vi "test_vi_new.vi"(5 "OutputReport_in":u8[](array[numeric]), 6 "DevDet_in":i32, 7 "InputReport_in":u8[](array[numeric])) -> (0 "DevDet_out":i32, 1 "OutputReport_out":u8[](array[numeric]), 2 "InputReport_out":u8[](array[numeric]) format="%x", 3 "output param":string)   [LabVIEW 2022 SP3]
uses:
  adcDLL_0001.dll
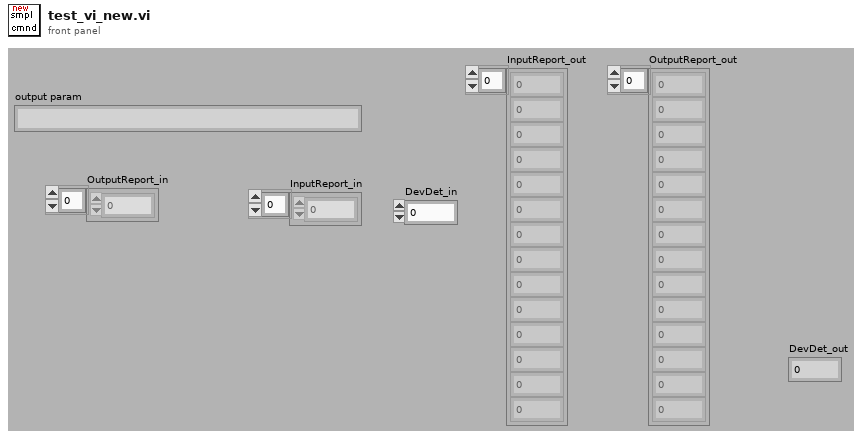
[diagram p1: front panel]
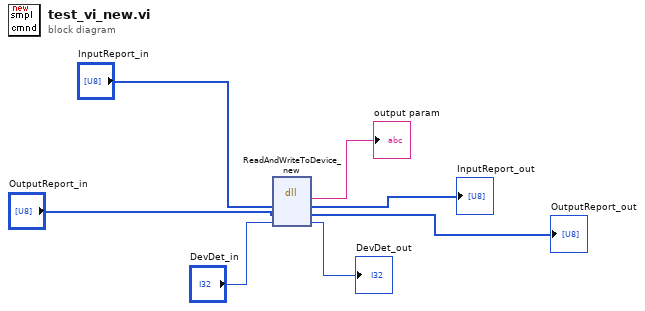
[diagram p0: block diagram]
diagram:
  n1 = dll-call lib="D:/LabVIEWSuite_64_OS/Spectrometers/ASEQ LR1/adcDLL_0001.dll" fn="ReadAndWriteToDevice_new"("InputReport1"="InputReport_in", "OutputReport1"="OutputReport_in", "DevDet"="DevDet_in") -> ("return type"=→"output param":string, "InputReport1"=→"InputReport_out":u8[], "OutputReport1"=→"OutputReport_out":u8[], "DevDet"=→"DevDet_out":i32)  [unwired: 3 in, 2 out]
